vi "closeJob.vi"(8 "error in (no error)":errorcluster, 11 "Job in":refnum<class "Job.lvclass">) -> (0 "error out":errorcluster, 3 "Job out":refnum<class "Job.lvclass">)   [LabVIEW 2013, in "openCronJob.lvlib" / "Job.lvclass"]
uses:
  Job.lvclass
  Job Details -- cluster.ctl
  Job.lvclass/Job.ctl
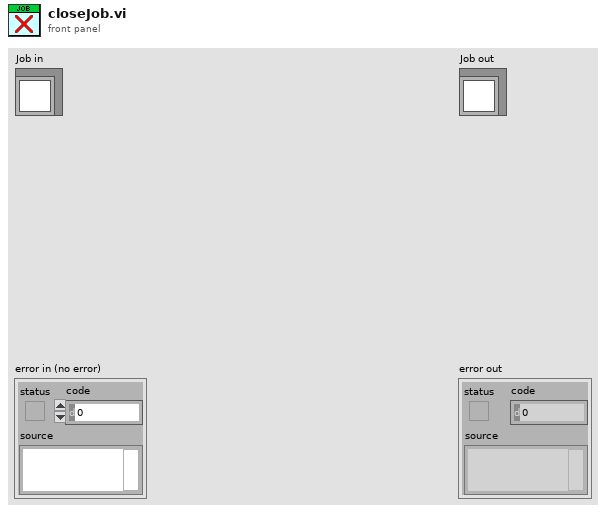
[diagram p1: front panel]
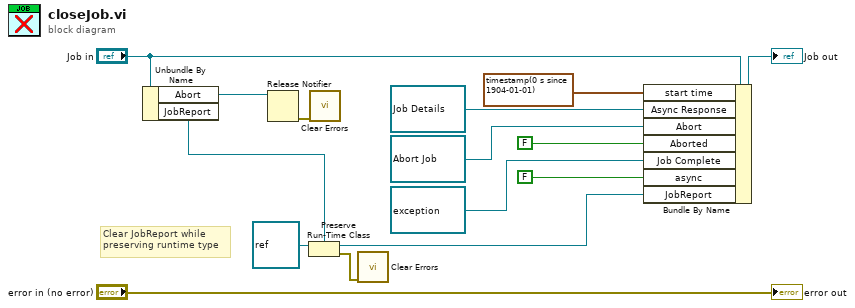
[diagram p0: block diagram]
diagram:
  # "Clear JobReport while\npreserving runtime type"
  n1 = Unbundle By Name("Job in") -> ("Abort"=w9:refnum<notifier>, "JobReport"=w3:refnum<class "JobReport.lvclass">)
  n2 = Release Notifier(notifier=w9) -> (error out=w12:errorcluster)  [unwired: 2 in, 2 out]
  n3 = Preserve Run-Time Class(object in=refnum<class> refnum, 2:w3) -> (object out=w2:refnum<class "JobReport.lvclass">, error out=w1:errorcluster)  [unwired: 1 in]
  n4 = call <vilib>:"Clear Errors.vi"("error in (no error)"=w12) -> ()  [unwired: 6 in, 1 out]
  n5 = call <vilib>:"Clear Errors.vi"("error in (no error)"=w1) -> ()  [unwired: 6 in, 1 out]
  n6 = Bundle By Name(cluster="Job in", "start time"=timestamp(0 s since 1904-01-01), "Async Response"=refnum<notifier> refnum, "Abort"=refnum<notifier> refnum, "Aborted"=FALSE, "Job Complete"=refnum<notifier> refnum, "async"=FALSE, "JobReport"=w2) -> (→"Job out":refnum<class "Job.lvclass">)
  "error out" <- "error in (no error)"
